vi "BlueSerializableClassName.vi"() -> (3 "BlueSerialization.lvlib:BlueSerializable.lvclass":string)   [LabVIEW 2020, in "BlueSerialization.lvlib" / "BlueSerializer.lvclass"]
uses:
  BlueSerializer.lvclass
  BlueSerializable/BlueSerializable.lvclass
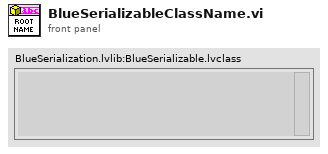
[diagram p1: front panel]
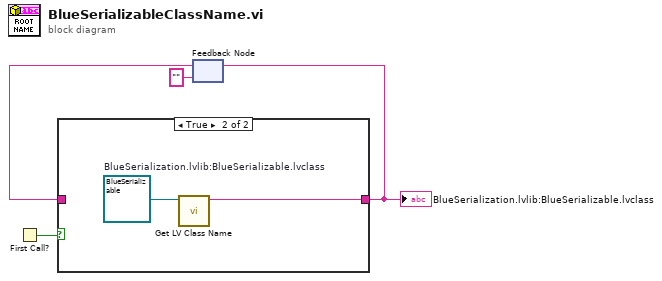
[diagram p0: block diagram]
diagram:
  n1 = First Call?() -> (First Call?: T/F=w4:bool)
  n2 = feedback #1("" ("class name")) -> (w1:string)
  n3 = case shown="True" w4 {
    tunnel: [w5 w6] -> w3
    tunnel: w1 -> [w5 _]
    frame False {
    }
    frame True {
      w7 = refnum<class "BlueSerializable.lvclass"> refnum  # BlueSerialization.lvlib:BlueSerializable.lvclass
      n4 = call <vilib>:"Get LV Class Name.vi"("object"=w7) -> ("class name"=w6:string)  [unwired: 9 in, 1 out]
    }
  }
  "BlueSerialization.lvlib:BlueSerializable.lvclass" <- w3
  n5 = feedback-in #1(w3) -> ()
